vi "LUnit API.vi"() -> ()   [LabVIEW 2020]
uses:
  <vilib>/Astemes/LUnit/LUnit Execution API.lvclass
panel:
  out "Output":string
  out "Test Time [ms]":u32
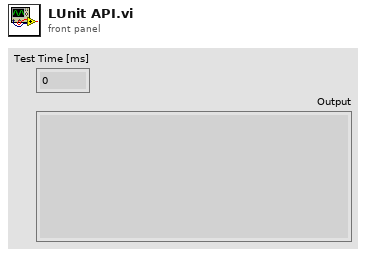
[diagram p1: front panel]
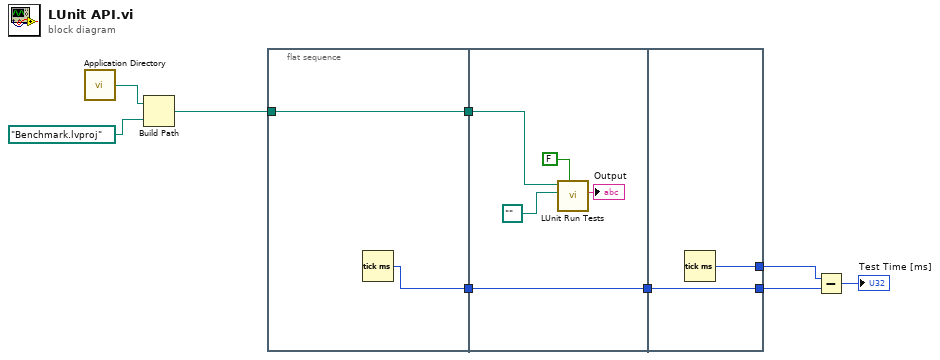
[diagram p0: block diagram]
diagram:
  n1 = call <vilib>:"Application Directory.vi"() -> ("Application Directory"=w9:path)
  n2 = Build Path(base path=w9, name or relative path=path "Benchmark.lvproj" ("Path")) -> (appended path=w1:path)
  n3 = flat-sequence {
    tunnel: [w11] -> w7
    tunnel: w1 -> [w11]
    tunnel: [w10] -> w5
    tunnel: w7 -> [w16]
    tunnel: w5 -> [w13]
    tunnel: [w13] -> w4
    tunnel: [w18] -> w6
    tunnel: w4 -> [w17]
    tunnel: [w17] -> w3
    frame #0 {
      n4 = Tick Count (ms)() -> (millisecond timer value=w10:u32)
    }
    frame #1 {
      n5 = call <vilib>:"LUnit Run Tests.vi"("Run Tests In Parallel? (T)"=FALSE, "Report Output path"=path "", "Project, Library, or Test Class Path"=w16) -> ("Output"=→"Output":string)  [unwired: 7 in, 1 out]
    }
    frame #2 {
      n6 = Tick Count (ms)() -> (millisecond timer value=w18:u32)
    }
  }
  n7 = Subtract(x=w6, y=w3) -> (x-y=→"Test Time [ms]":u32)
